vi "Strip Path to exe.vi"(11 "File Path Control":path=path "D:/MMU Control/Source_Code/LoadPLUS GUI/Builds/Executable/LoadPLUS.exe/LoadPLUS GUI/GUI/Misc/Version Information/Get LoadPlus Version.vi") -> (3 "Path to Exe":path)   [LabVIEW 2014]
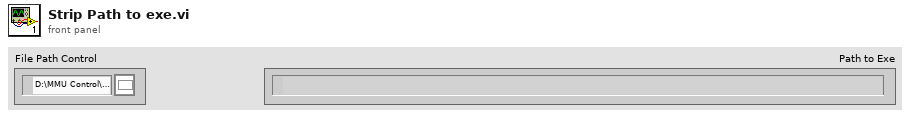
[diagram p1: front panel]
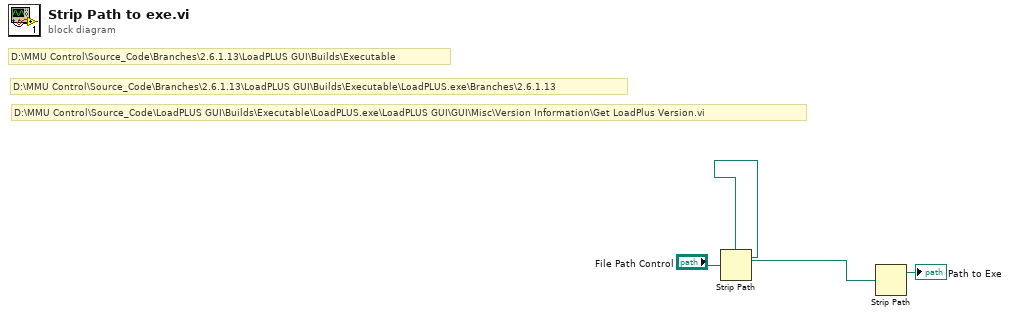
[diagram p0: block diagram]
diagram:
  # "D:\\MMU Control\\Source_Code\\Branches\\2.6.1.13\\LoadPLUS GUI\\Builds\\Executable"
  # "D:\\MMU Control\\Source_Code\\Branches\\2.6.1.13\\LoadPLUS GUI\\Builds\\Executable\\LoadPLUS.exe\\Branches\\2.6.1.13"
  # "D:\\MMU Control\\Source_Code\\LoadPLUS GUI\\Builds\\Executable\\LoadPLUS.exe\\LoadPLUS GUI\\GUI\\Misc\\Version Information\\Get LoadPlus Version.vi"
  n1 = Strip Path(path="File Path Control") -> (stripped path=w1:path)  [unwired: 1 out]
  n2 = Strip Path(path=w1) -> (stripped path=→"Path to Exe":path)  [unwired: 1 out]
